vi "Reverse Polish Notation.vi"() -> ()   [LabVIEW 2013]
panel:
  in  "Equals":bool
  in  "Backspace":bool
  in  "Clear":bool
  in  "Multiply":bool
  in  "Divide":bool
  in  "Minus":bool
  in  "Plus":bool
  in  "Space":bool
  in  "Button 0":bool
  in  "Button 9":bool
  in  "Button 8":bool
  in  "Button 7":bool
  in  "Button 6":bool
  in  "Button 5":bool
  in  "Button 4":bool
  in  "Button 3":bool
  in  "Button 2":bool
  in  "Button 1":bool
  out "Display":string
  # "TI-90+ Silver Edition"
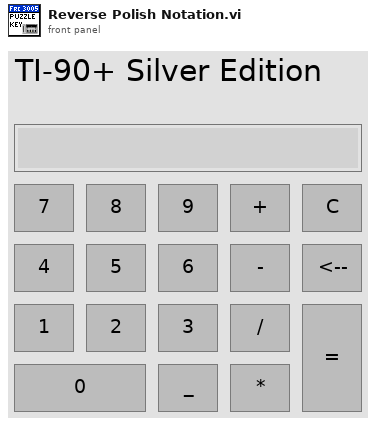
[diagram p1: front panel]
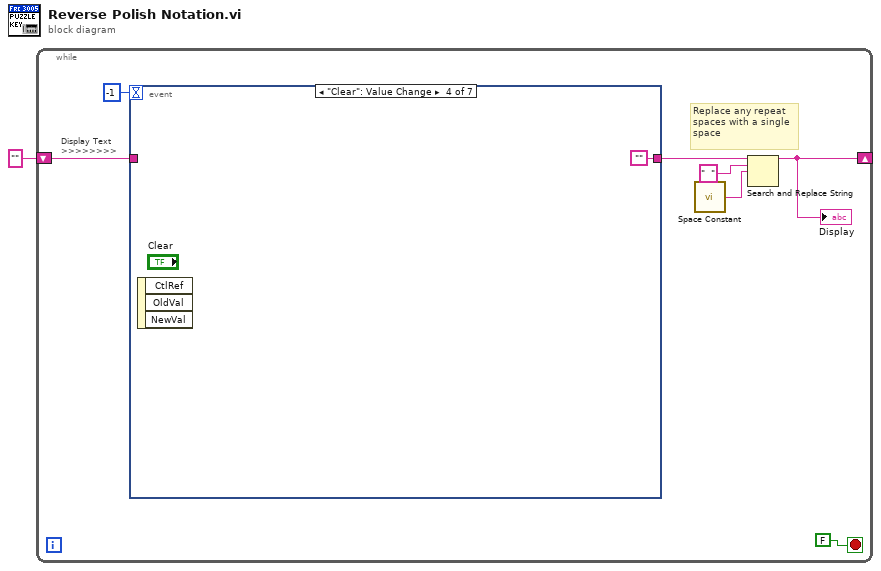
[diagram p0: block diagram]
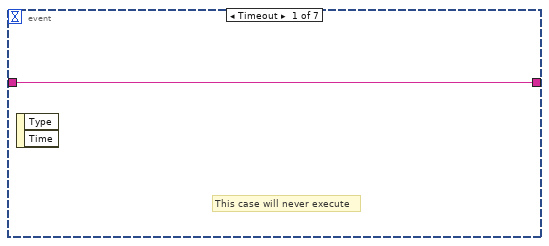
[diagram p2: hidden frame]
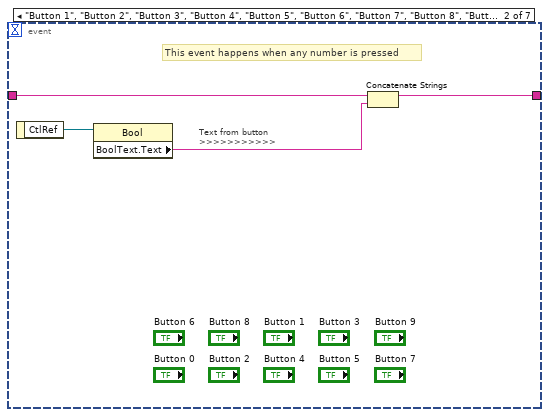
[diagram p3: hidden frame]
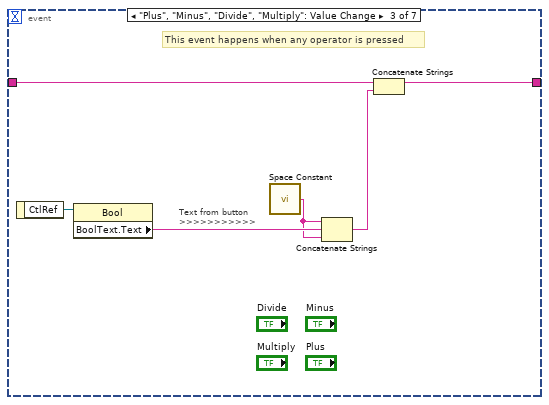
[diagram p4: hidden frame]
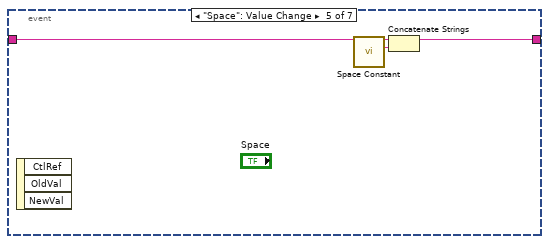
[diagram p5: hidden frame]
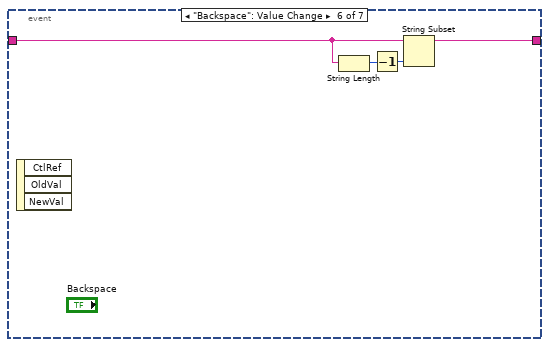
[diagram p6: hidden frame]
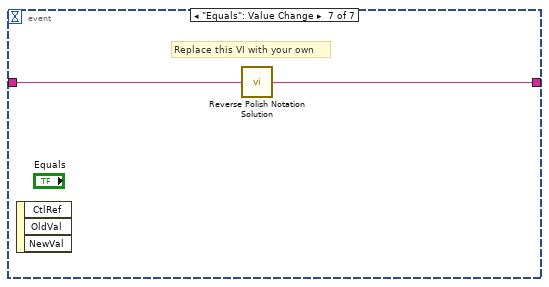
[diagram p7: hidden frame]
diagram:
  n1 = while {
    shift-right: [w2] -> _
    shift-left: "" ("Display") -> [w6]
    stop <- FALSE stop-if-true
    # "Replace any repeat\nspaces with a single\nspace"
    # "Display Text\n>>>>>>>>"
    n2 = event shown="[3] \"Clear\": Value Change" {
      selector: _ -> [_ _ _ _ _ _ _]
      dyn-events: _ -> [_ _ _ _ _ _ _]
      timeout: -1 -> [_ _ _ _ _ _ _]
      tunnel: w6 -> [w9 w12 w16 _ w22 w26 w28]
      tunnel: [w9 w11 w14 "" w23 w27 w29] -> w3
      event Timeout {
        # "This case will never execute"
        n3 = event-data() -> ()  [unwired: 1 in, 2 out]
      }
      event "Button 1", "Button 2", "Button 3", "Button 4", "Button 5", "Button 6", "Button 7", "Button 8", "Button 9", "Button 0": Value Change {
        # "Text from button\n>>>>>>>>>>>"
        # "This event happens when any number is pressed"
        n4 = event-data() -> ("CtlRef"=w13:refnum<vi>)  [unwired: 1 in]
        n5 = property class="Bool"(reference=w13) -> ("BoolText.Text"=w10:string)  [unwired: 1 in, 2 out]
        n6 = Concatenate Strings(w12, w10) -> (w11:string)
      }
      event "Plus", "Minus", "Divide", "Multiply": Value Change {
        # "Text from button\n>>>>>>>>>>>"
        # "This event happens when any operator is pressed"
        n7 = event-data() -> ("CtlRef"=w19:refnum<vi>)  [unwired: 1 in]
        n8 = property class="Bool"(reference=w19) -> ("BoolText.Text"=w18:string)  [unwired: 1 in, 2 out]
        n9 = call <vilib>:"Space Constant.vi"() -> ("String"=w15:string)
        n10 = Concatenate Strings(w15, w18, w15) -> (w17:string)
        n11 = Concatenate Strings(w16, w17) -> (w14:string)
      }
      event "Clear": Value Change {
        n12 = event-data() -> ()  [unwired: 1 in, 3 out]
      }
      event "Space": Value Change {
        n13 = event-data() -> ()  [unwired: 1 in, 3 out]
        n14 = call <vilib>:"Space Constant.vi"() -> ("String"=w21:string)
        n15 = Concatenate Strings(w22, w21) -> (w23:string)
      }
      event "Backspace": Value Change {
        n16 = event-data() -> ()  [unwired: 1 in, 3 out]
        n17 = String Length(string=w26) -> (length=w24:i32)
        n18 = Decrement(x=w24) -> (x-1=w25:i32)
        n19 = String Subset(string=w26, length (rest)=w25) -> (substring=w27:string)  [unwired: 1 in]
      }
      event "Equals": Value Change {
        # "Replace this VI with your own"
        n20 = event-data() -> ()  [unwired: 1 in, 3 out]
        n21 = call "Reverse Polish Notation Solution.vi"("Input"=w28) -> ("Output"=w29:string)
      }
    }
    n22 = call <vilib>:"Space Constant.vi"() -> ("String"=w4:string)
    n23 = Search and Replace String(input string=w3, search string="  ", replace string=w4) -> (result string=w2:string)  [unwired: 5 in, 3 out]
    "Display" <- w2
  }
